vi "擦除OOC.vi"(8 "error in":errorcluster) -> (0 "error out":errorcluster, 2 "return":i32)   [LabVIEW 2016]
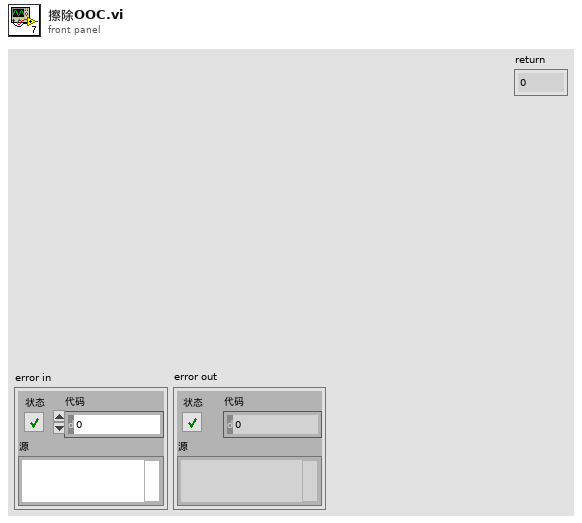
[diagram p1: front panel]
types:
  T1 = cluster{"byCmdType":u8, "bySubCmd":u8, "byPara":u8, "byAddr_h":u8, "byAddr_l":u8, "byAddr_ll":u8, "byLen_h":u8, "byLen_l":u8}
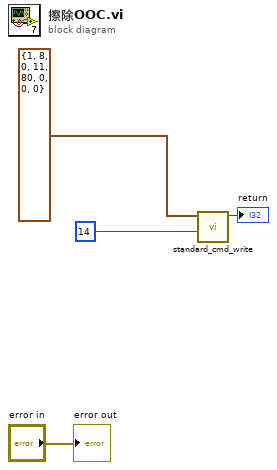
[diagram p0: block diagram]
diagram:
  n1 = call "standard_cmd_write.vi"("dwLen"=u32 14, "cmd_std_header_t"=T1 {"byCmdType"=1, "bySubCmd"=8, "byPara"=0, "byAddr_h"=11, "byAddr_l"=80, "byAddr_ll"=0, "byLen_h"=0, "byLen_l"=0}) -> ("return"=→"return":i32)  [unwired: 9 in]
  "error out" <- "error in"
